vi "Check Data Model.vi"(8 "error in":errorcluster, 11 "device data model in":refnum<class "Device Data Model.lvclass">) -> (0 "error out":errorcluster, 3 "device data model out":refnum<class "Device Data Model.lvclass">)   [LabVIEW 2012, in "Device Data Model.lvclass"]
doc: "This VI ensures that the data model has at least 65,535 values of every type. This is required for certain modbus function codes."
uses:
  Device Data Model.lvclass
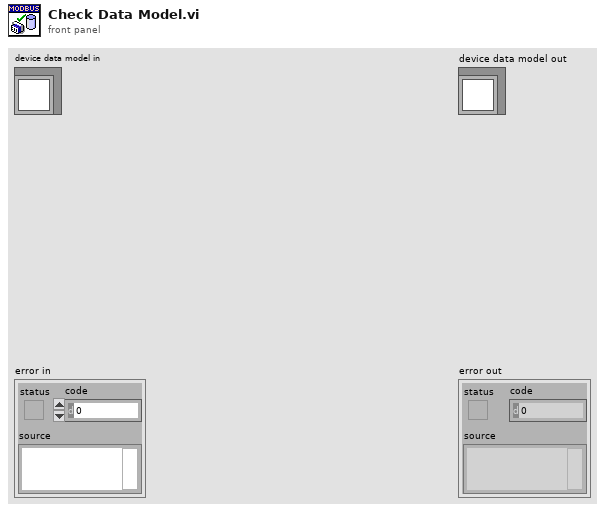
[diagram p1: front panel]
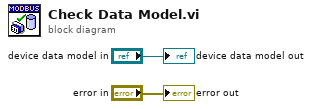
[diagram p0: block diagram]
diagram:
  "error out" <- "error in"
  "device data model out" <- "device data model in"
